vi "backup.vi"() -> ()   [LabVIEW 2017]
uses:
  <vilib>/myRIO/Instrument Drivers/Utilities/Utilities.lvlib
  qsm/type defs/states.ctl
  qsm/type defs/action buttons.ctl
panel:
  in  "action buttons":T1
  out "y0 (circle)":i32
  out "x0 (circle)":i32
  out "x1 (circle)":i32
  out "y1 (circle)":i32
  in  "divider (circle)":sgl=1.0
  out "Radius (circle)":dbl
  out "Circles Calibrated (Shape Detection 1)":T2(array[cluster]) {"Position"."Y" format="%.2f"; "Position"."X" format="%.2f"}
  in  "ROI Descriptor COLOR Mask":T3={"Global Rectangle"=[0, 0, 0, 0], "Contours"=[{"ID"=enum."External", "Type"=0, "Coordinates"=[0, 0, 0, 0]}]}
  in  "ROI Descriptor (COLOR Mask 1)":T3={"Global Rectangle"=[51, 157, 345, 350], "Contours"=[{"ID"=enum."External", "Type"=5, "Coordinates"=[137, 230, 93, 226, 75, 199, 49, 200, 56, 145, 98, 111, 200, 119, 250, 126, 235, 166, 240, 212, 188, 243, 303, 244, 336, 247, 336, 271, 335, 292, 335, 318, 314, 323, 293, 334, 279, 345, 272, 349, 187, 349, 186, 335, 120, 334, 112, 314, 100, 297, 59, 291, 51, 288, 51, 287]}]} {"Contours"."Type" items=["No Selection", "Point", "Line", "Rectangle", "Oval", "Polygon", "Freehand Region", "Annulus", "Unused2", "Unused3", "Broken Line", "Freehand Line", "Rotated Rectangle"]}
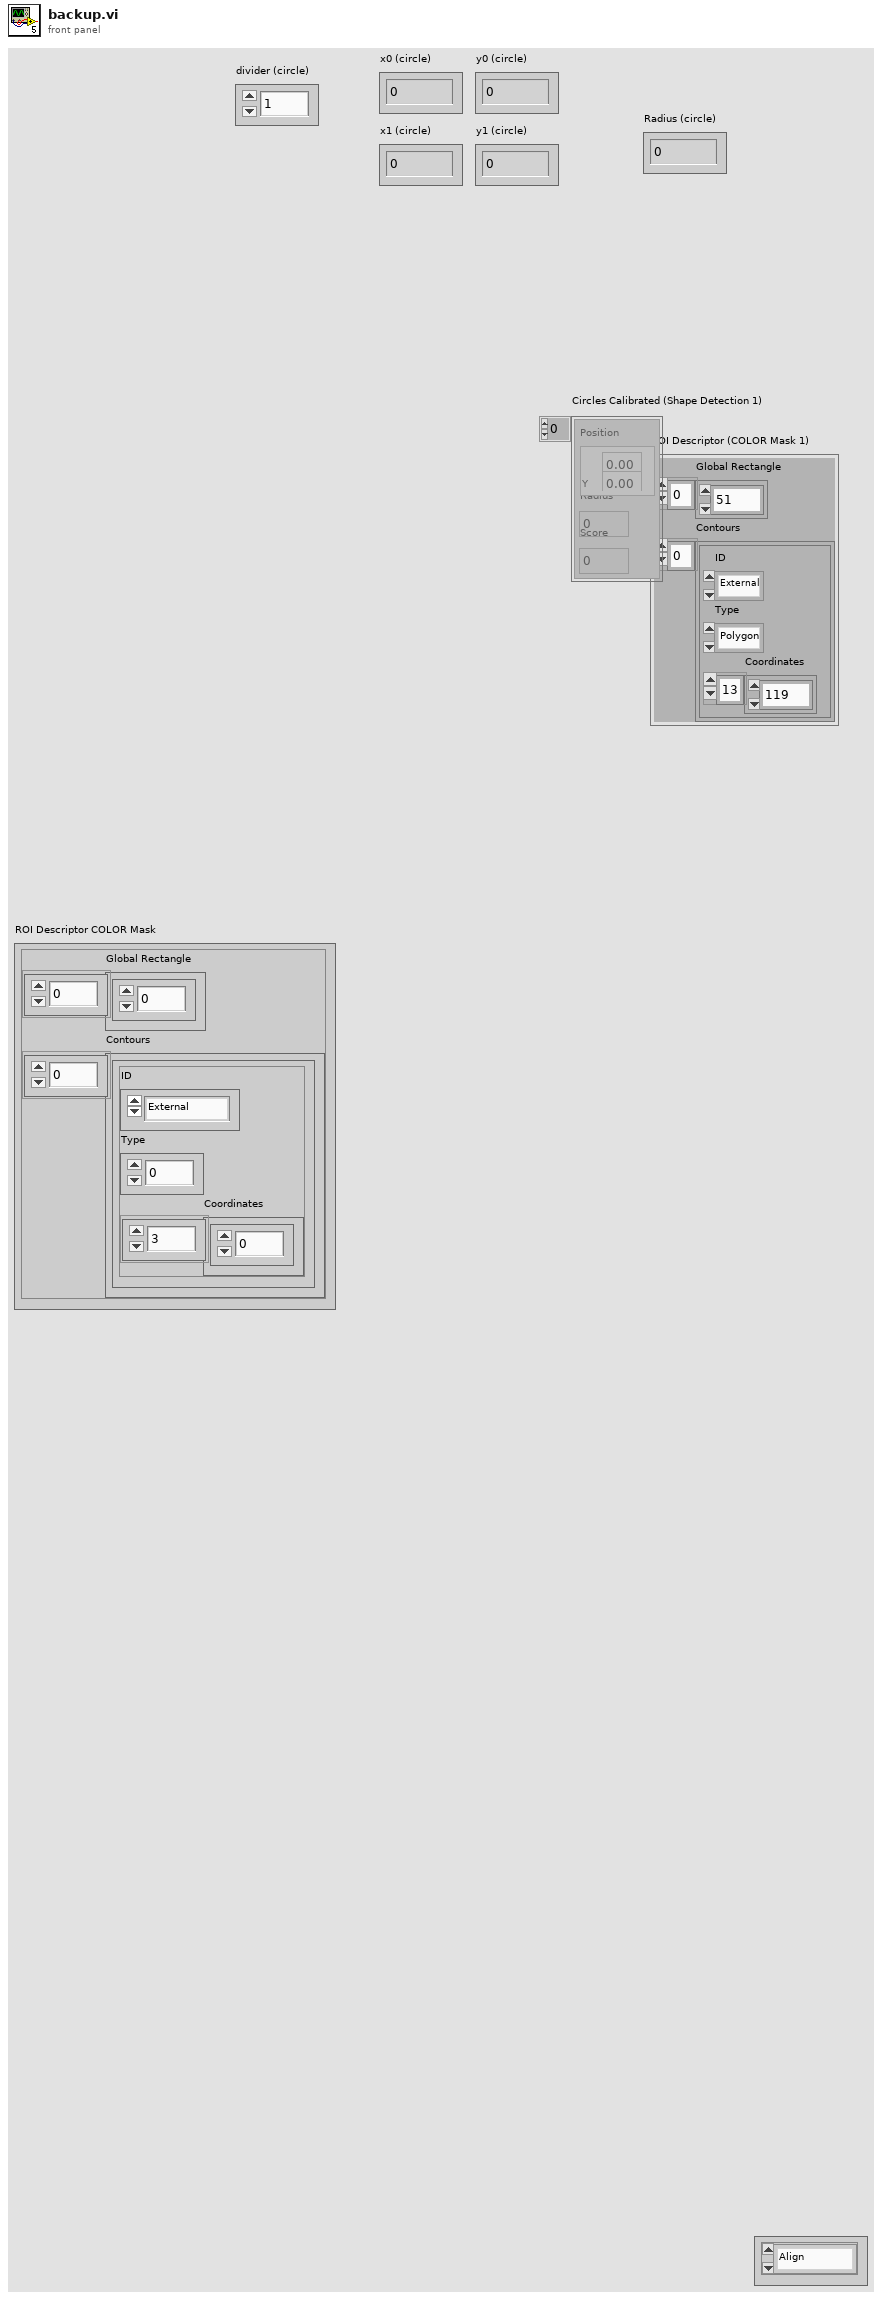
[diagram p1: front panel]
types:
  T1 = typedef "action buttons.ctl" = cluster{"Shape - t, Color - f":enum16{"Align", "Pattern", "Ball", "Other", "Clear", "Joystick control"}}
  T2 = cluster{"Position":cluster{"X":sgl, "Y":sgl}, "Radius":dbl, "Score":dbl}[]
  T3 = cluster{"Global Rectangle":i32[], "Contours":cluster{"ID":enum32{"External", "Internal"}, "Type":u32, "Coordinates":i32[]}[]}
  T4 = typedef "states.ctl" = enum16{"(qsm) schedule", "(qsm) initialize", "(qsm) release", "(qsm) clean up", "(qsm) shutdown", "(myRIO) initialize", "(myRIO) clean up", "(myRIO) update ports", "(image) get", "(image) analyze", "(image) overlay", "(image) show", "save image", "(ball) Shape detection", "(ball) Calculate ROI", "X align", "Y align", "Wait", "Grab", "(pattern) Find Square", "(pattern) Calculate ROI", "(pattern) Analyze pattern", "Compare", "(joystick) Joystick X, manip's", "(joystick) Joystick Y", "Wait for button"}
  T5 = cluster{"Position":cluster{"X":sgl, "Y":sgl}, "Radius":dbl, "Score":dbl}
  T6 = cluster{"ID":enum32{"External", "Internal"}, "Type":u32, "Coordinates":i32[]}[]
  T7 = cluster{"ID":enum32{"External", "Internal"}, "Type":u32, "Coordinates":i32[]}
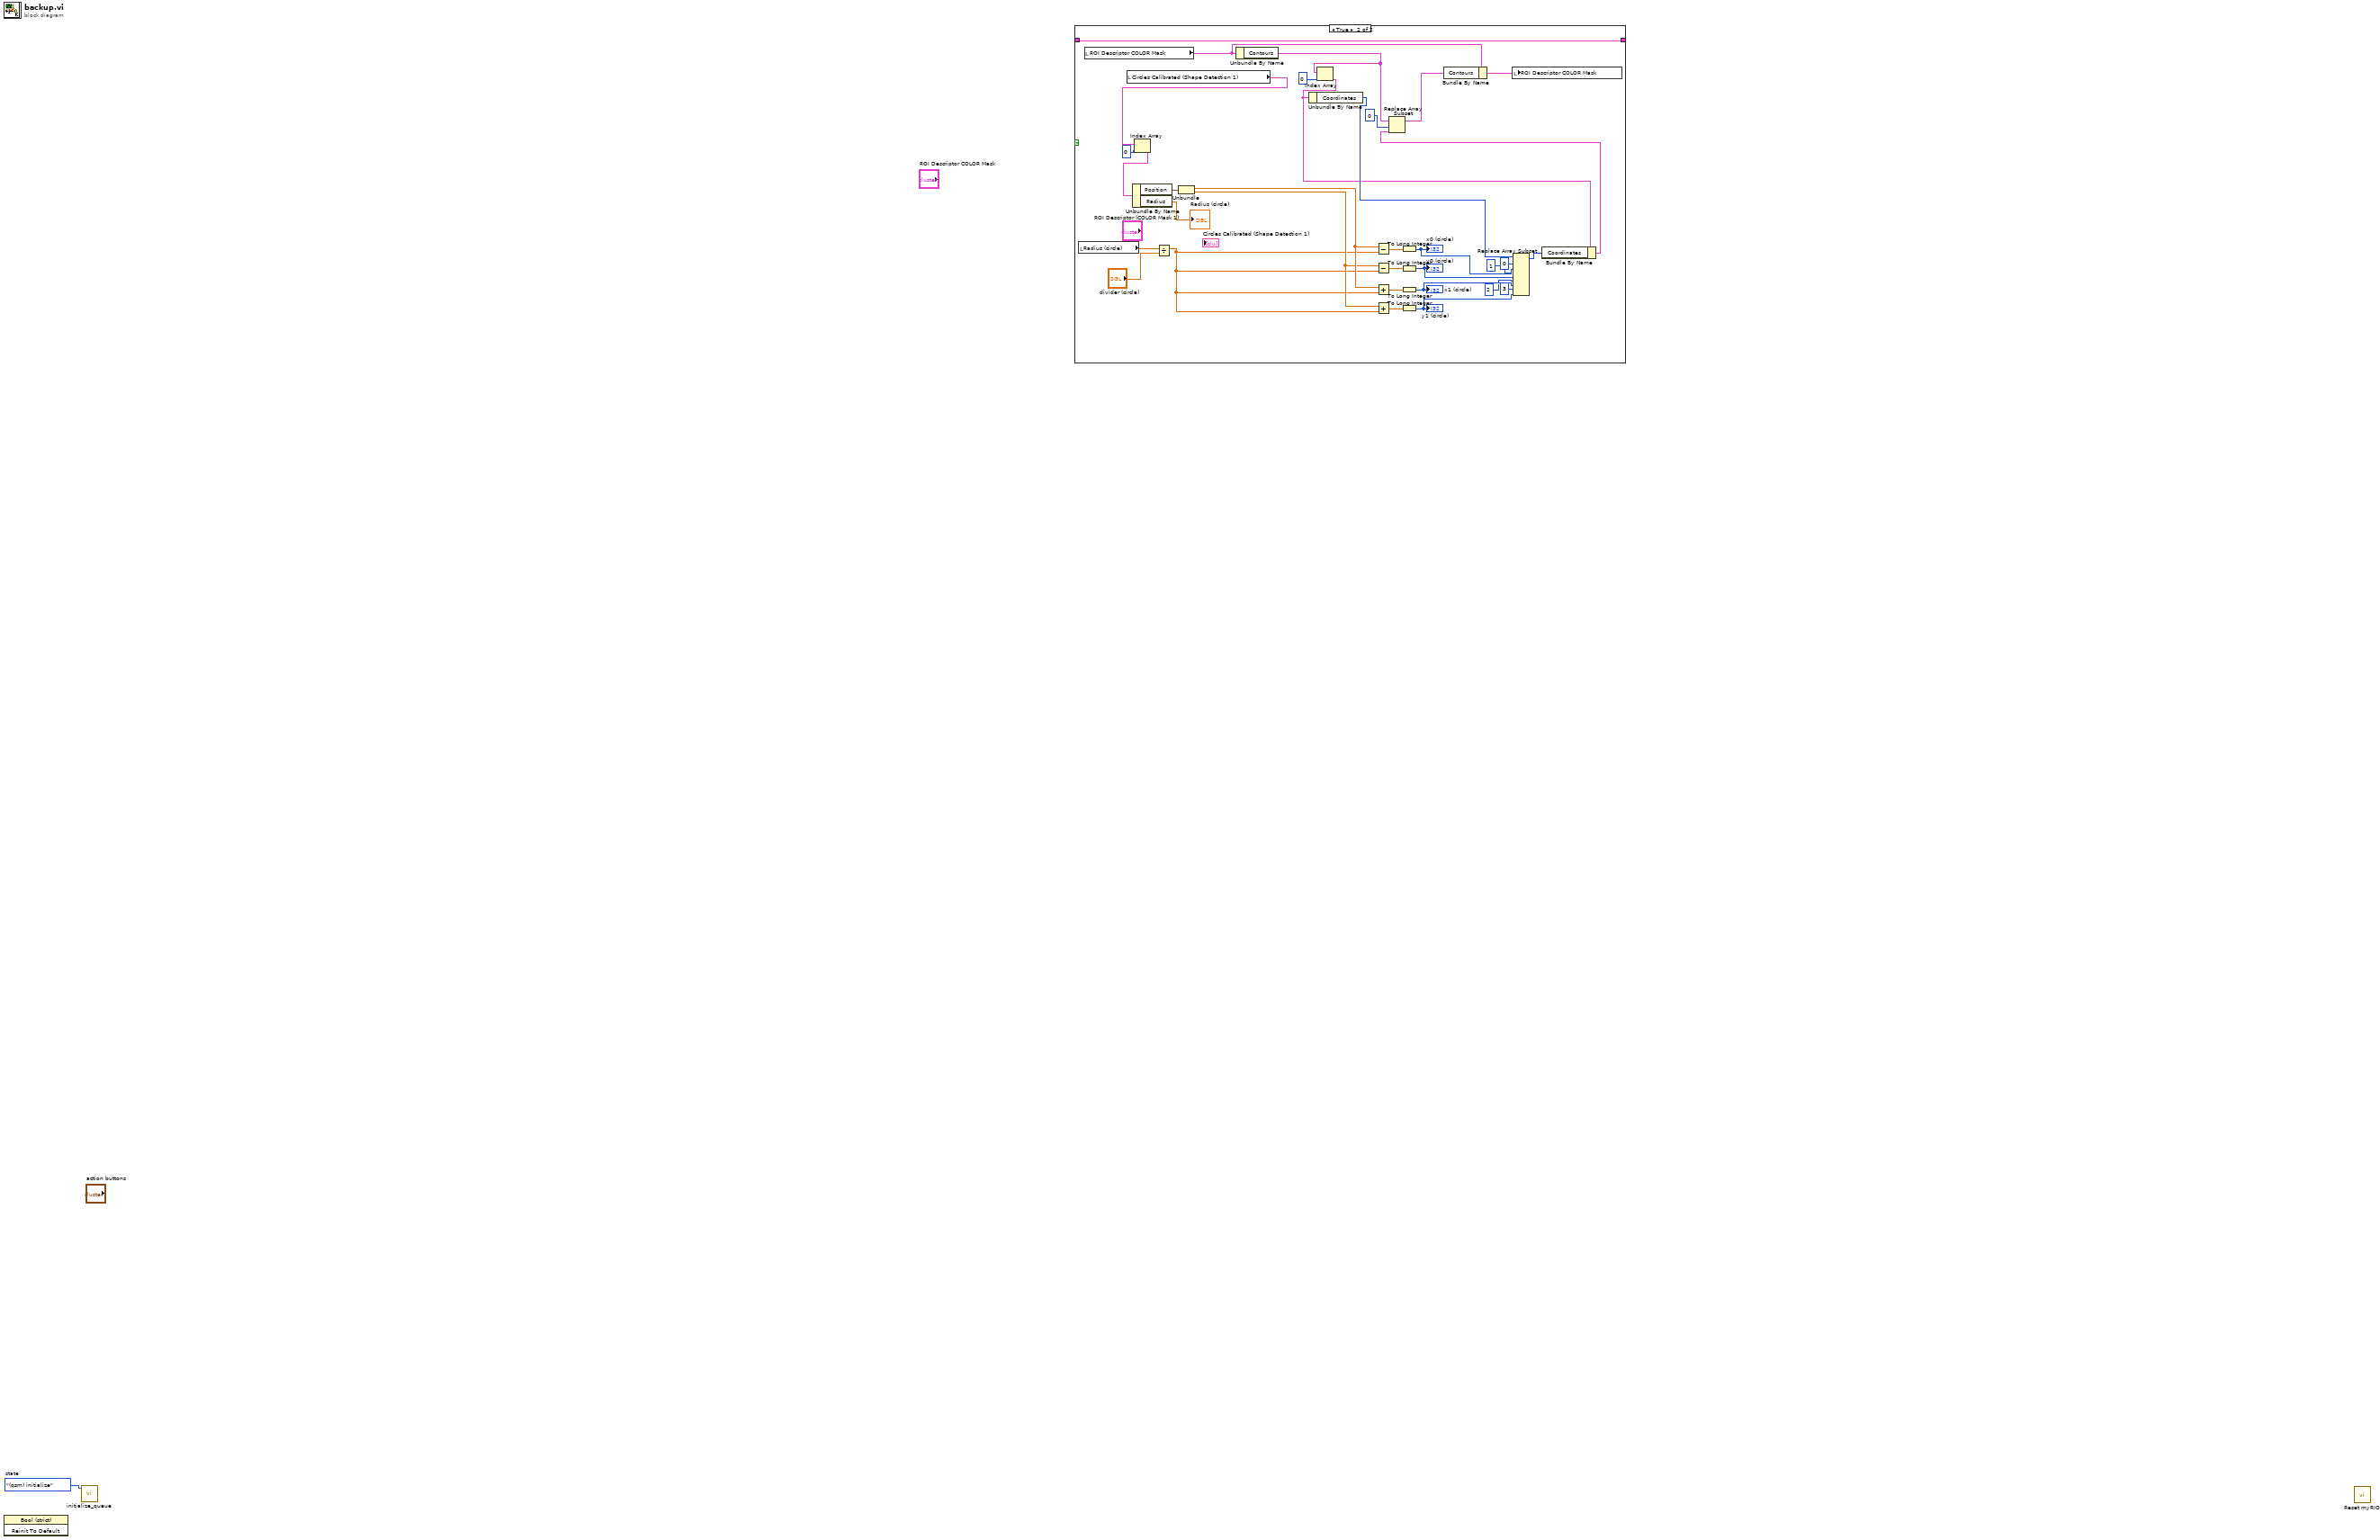
[diagram p0: block diagram]
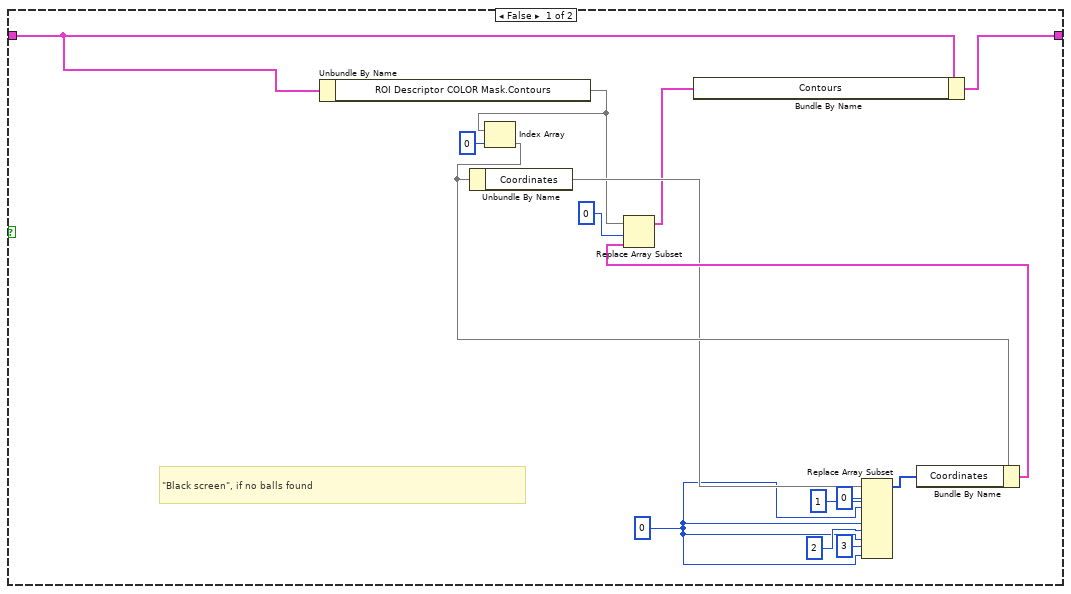
[diagram p2: hidden frame]
diagram:
  w1 = states."(qsm) initialize"  # state
  n1 = invoke on="Invoke Node" class="Bool (strict)" method="Reinit To Default"() -> ()  [unwired: 3 in, 3 out]
  n2 = call "initialize_queue.vi"("state"=w1) -> ("error out"=w2:errorcluster, "queue out"=w3:refnum<queue>)  [unwired: 9 in]
  n3 = case shown="True" {
    selector: _ -> [_ _]
    tunnel: [w7 w21] -> _
    tunnel: _ -> [w6 w21]
    frame False {
      w8 = 0 ("index")
      # "\"Black screen\", if no balls found"
      n4 = Unbundle By Name(w6) -> ("ROI Descriptor COLOR Mask.Contours"=w15)
      n5 = Index Array(array=w15, index=0) -> (element=w18)
      n6 = Unbundle By Name(w18) -> ("Coordinates"=w17)
      n7 = Replace Array Subset(array=w17, new element #1=w8, index #1=0 ("index"), new element #2=w8, index #2=1 ("index"), new element #3=w8, index #3=2 ("index"), new element #4=w8, index #4=3 ("index")) -> (w19:i32[])
      n8 = Bundle By Name(cluster=w18, "Coordinates"=w19) -> (w20:cluster{})
      n9 = Replace Array Subset(array=w15, new element=w20, index=0) -> (w16:cluster{}[])
      n10 = Bundle By Name(cluster=w6, "Contours"=w16) -> (w7:cluster{})
    }
    frame True {
      n11 = local read "Radius (circle)"() -> (w28:dbl)
      n12 = local read "ROI Descriptor COLOR Mask"() -> (w23:T3)
      n13 = local read "Circles Calibrated (Shape Detection 1)"() -> (w53:T2)
      n14 = Index Array(array=w53, index=0) -> (element=w51:T5)
      n15 = Unbundle By Name(w51) -> ("Position"=w50:cluster{"X":sgl, "Y":sgl}, "Radius"=→"Radius (circle)":dbl)
      n16 = Divide(x=w28, y="divider (circle)") -> (x/y=w27:dbl)
      n17 = Unbundle(w50) -> ("X"=w47:sgl, "Y"=w46:sgl)
      n18 = Unbundle By Name(w23) -> ("Contours"=w25:T6)
      n19 = Index Array(array=w25, index=0) -> (element=w39:T7)
      n20 = Unbundle By Name(w39) -> ("Coordinates"=w41:i32[])
      n21 = Subtract(x=w47, y=w27) -> (x-y=w45:dbl)
      n22 = Subtract(x=w46, y=w27) -> (x-y=w44:dbl)
      n23 = Add(x=w47, y=w27) -> (x+y=w42:dbl)
      n24 = Add(x=w46, y=w27) -> (x+y=w43:dbl)
      n25 = To Long Integer(number=w45) -> (32bit integer=w36:i32)
      "x0 (circle)" <- w36
      n26 = To Long Integer(number=w44) -> (32bit integer=w35:i32)
      "y0 (circle)" <- w35
      n27 = To Long Integer(number=w42) -> (32bit integer=w34:i32)
      "x1 (circle)" <- w34
      n28 = To Long Integer(number=w43) -> (32bit integer=w33:i32)
      "y1 (circle)" <- w33
      n29 = Replace Array Subset(array=w41, new element #1=w36, index #1=0 ("index"), new element #2=w35, index #2=1 ("index"), new element #3=w34, index #3=2 ("index"), new element #4=w33, index #4=3 ("index")) -> (w38:i32[])
      n30 = Bundle By Name(cluster=w39, "Coordinates"=w38) -> (w37:T7)
      n31 = Replace Array Subset(array=w25, new element=w37, index=0) -> (w22:T6)
      n32 = Bundle By Name(cluster=w23, "Contours"=w22) -> (w24:T3)
      n33 = local write "ROI Descriptor COLOR Mask"(w24) -> ()
    }
  }
  n34 = call <vilib>:"Reset myRIO.vi"() -> ("error in (no error)"=w5:errorcluster)  [unwired: 10 in, 1 out]
